vi "clearerror.vi"(8 "error in (no error)":errorcluster, 11 "Clear Error":bool) -> (0 "error out":errorcluster)   [LabVIEW 2018, in "pid-toolkit.lvlib"]
uses:
  pid-toolkit.lvlib
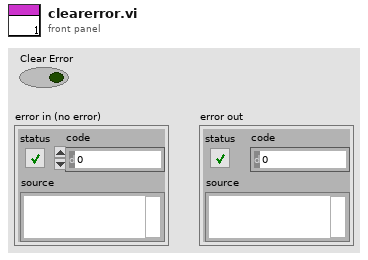
[diagram p1: front panel]
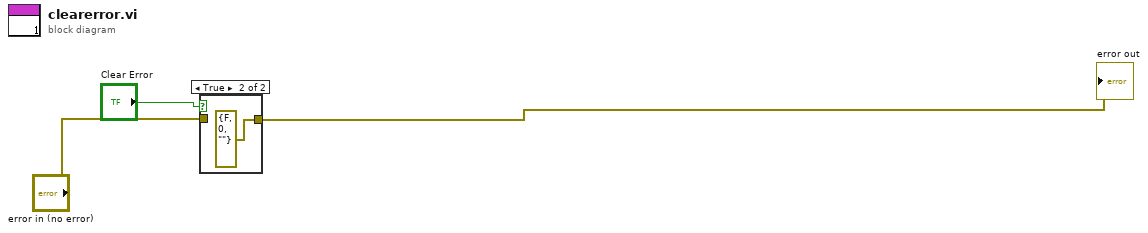
[diagram p0: block diagram]
diagram:
  n1 = case shown="True" "Clear Error" {
    tunnel: "error in (no error)" -> [w4 _]
    tunnel: [w4 errorcluster {"status"=FALSE, "code"=0, "source"=""} ("Modbus error")] -> w2
    frame False {
    }
    frame True {
    }
  }
  "error out" <- w2
